vi "Start Autodiscover Group.vi"(8 "error in (no error)":errorcluster, 10 "Discovery":T1, 11 "RemoteDataService in":refnum<class "RemoteDataService.lvclass">) -> (0 "error out":errorcluster, 3 "RemoteDataService out":refnum<class "RemoteDataService.lvclass">)   [LabVIEW 2020, in "Vecto.lvlib" / "RemoteDataService.lvclass"]
uses:
  RemoteDataService.lvclass
  lv-volatus/messages/Discovery/Data.ctl
  lv-volatus/messages/Service/Data.ctl
  lv-volatus/messages/ServiceType/Enumeration.ctl
  Autodiscover Group Async.vi
  RemoteDataService.lvclass/RemoteDataService.ctl
  lv-volatus/messages/ServiceType/ServiceType.lvlib
  lv-volatus/messages/Service/Service.lvlib
  lv-volatus/messages/Discovery/Discovery.lvlib
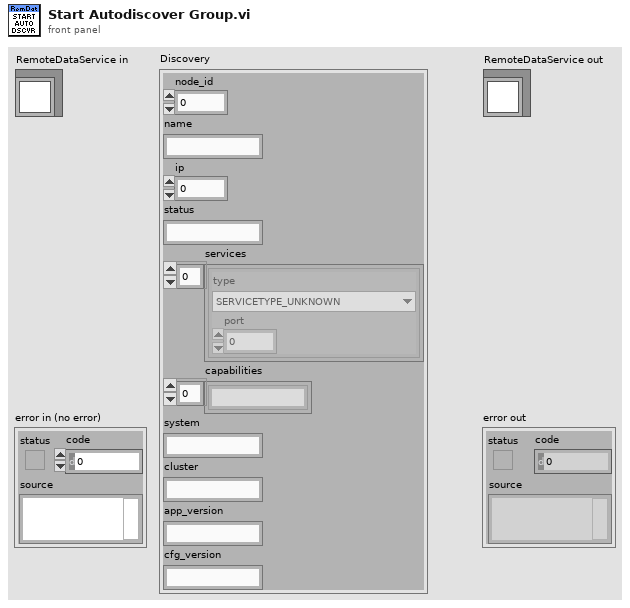
[diagram p1: front panel]
types:
  T1 = typedef "Discovery.lvlib/Data.ctl" = cluster{"node_id":u32, "name":string, "ip":u32, "status":string, "services":T2[], "capabilities":string[], "system":string, "cluster":string, "app_version":string, "cfg_version":string}
  T2 = typedef "Service.lvlib/Data.ctl" = cluster{"type":T3, "port":i32}
  T3 = typedef "ServiceType.lvlib/Enumeration.ctl" = enum16{"SERVICETYPE_UNKNOWN", "SERVICETYPE_TCPSERVER", "SERVICETYPE_HTTPSERVER"}
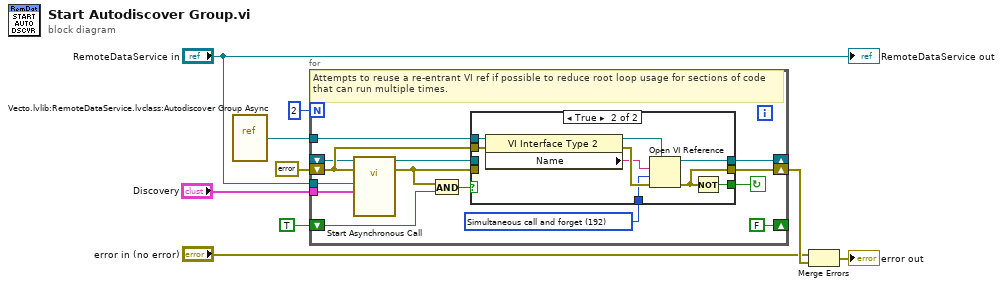
[diagram p0: block diagram]
diagram:
  n1 = vi-ref "Vecto.lvlib:RemoteDataService.lvclass:Autodiscover Group Async.vi"() -> (w9:refnum<vi>)
  n2 = for {
    N: 2 -> [_]
    tunnel: w9 -> [w22]
    shift-right: [w21] -> _
    shift-left: _ -> [w20]
    shift-right: [w18] -> w4
    shift-left: errorcluster {"status"=FALSE, "code"=0, "source"=""} ("error constant") -> [w23]
    shift-right: [FALSE] -> _
    shift-left: TRUE -> [w15]
    tunnel: "Discovery" -> [w11]
    tunnel: "RemoteDataService in" -> [w10]
    stop <- w14 continue-if-true
    w12 = 192 items=["Record modifications"=1, "Open templates for editing"=2, "Prompt user to save"=4, "Prepare for reentrant run"=8, "Prompt to find missing subVIs"=16, "Hide loading dialog box"=32, "Enable simultaneous calls"=64, "Prepare to call and forget"=128, "Simultaneous call and forget"=192, "Prepare to call and collect"=256, "Simultaneous call and collect"=320]
    # "Attempts to reuse a re-entrant VI ref if possible to reduce root loop usage for sections of code that can run multiple times."
    n3 = call-by-ref "Start Asynchronous Call"(reference=w20, error in=w23, "Discovery"=w11, "RemoteDataService in"=w10) -> (reference out=w19:refnum<vi>, error out=w17:errorcluster)  [unwired: 10 in]
    n4 = And(x=w17, y=w15) -> (x .and. y?=w16:bool)
    n5 = case shown="True" w16 {
      tunnel: w22 -> [_ w33]
      tunnel: w12 -> [_ w31]
      tunnel: [w25 w29] -> w21
      tunnel: w19 -> [w25 _]
      tunnel: [w24 w27] -> w18
      tunnel: w17 -> [w24 _]
      tunnel: w23 -> [_ w28]
      tunnel: [_ w26] -> w14
      frame False {
      }
      frame True {
        n6 = property class="VI Interface Type 2"(reference=w33, error in=w28) -> (reference out=w30:refnum<vi>, error out=w34:errorcluster, "Name"=w32:string)
        n7 = Open VI Reference(type specifier VI Refnum (for type only)=w30, vi path=w32, options=w31, error in (no error)=w34) -> (vi reference=w29:refnum<vi>, error out=w27:errorcluster)  [unwired: 2 in]
        n8 = Not(x=w27) -> (.not. x?=w26:bool)
      }
    }
  }
  n9 = Merge Errors("error in (no error)", w4) -> (→"error out":errorcluster)
  "RemoteDataService out" <- "RemoteDataService in"
